vi "Serialize as VTT.vi"(8 "error in (no error)":errorcluster, 11 "Data Item in":refnum<class "Data Item.lvclass">) -> (0 "error out":errorcluster, 2 "VTT Fragment":string, 3 "Data Item out":refnum<class "Data Item.lvclass">)   [LabVIEW 2020, in "VILab.lvlib" / "Data Item.lvclass"]
uses:
  Data Item.lvclass
  Data Item.lvclass/Data Item.ctl
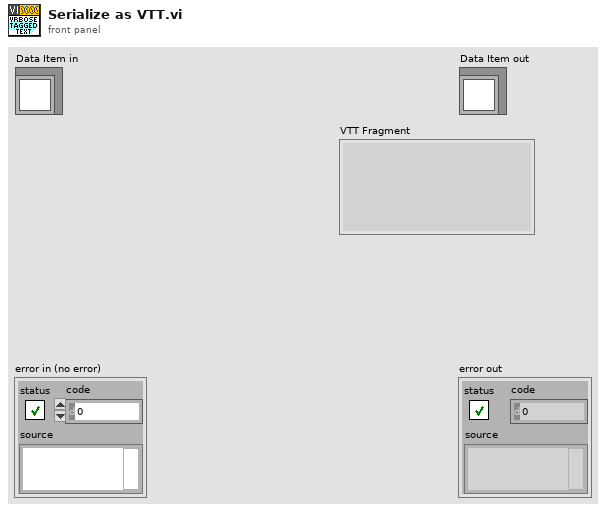
[diagram p1: front panel]
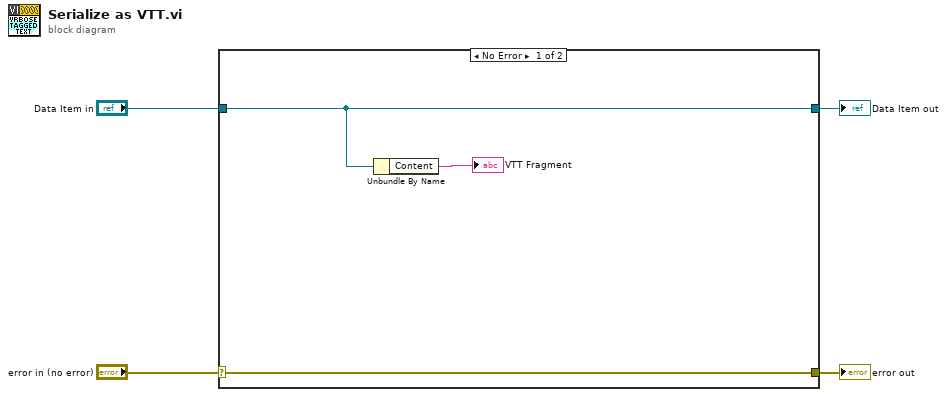
[diagram p0: block diagram]
diagram:
  n1 = case shown="No Error" "error in (no error)" {
    selector: "error in (no error)" -> [w5 w9]
    tunnel: [w5 w9] -> w3
    tunnel: [w7 w8] -> w1
    tunnel: "Data Item in" -> [w7 w8]
    frame No Error {
      n2 = Unbundle By Name(w7) -> ("Content"=→"VTT Fragment":string)
    }
    frame Error {
    }
  }
  "error out" <- w3
  "Data Item out" <- w1
